vi "TriWave1stEd_YNWang.vi"() -> ()   [LabVIEW 2014]
uses:
  <vilib>/Instr/_visa.llb/VISA Configure Serial Port (Instr).vi
panel:
  in  "Protect scan":bool
  out "Corrent Feedback":dbl
  out "XY Graph":cluster{dbl[], dbl[]}(graph)
  out "Feedback Current":dbl(graph)
  in  "VISA resource name":refnum<visa-resource-name>
  in  "Path":path
  out "Negative Scanning?":bool
  in  "Scan direction":bool
  out "Error":bool
  out "In pause state?":bool
  in  "Pause scan":bool
  in  "Wait before run/s":dbl
  out "Exception Thrown Panel":string
  in  "Emergent STOP":bool
  out "Output V":dbl format="%#_13g"
  in  "End V":dbl format="%#_13g"
  in  "Scan cycle":dbl format="%#_13g"
  out "Volt generator":dbl(graph)
  in  "Step Time/ms":dbl format="%#_13g"
  in  "V per step":dbl format="%#_13g"
  in  "Low V":dbl format="%#_13g"
  in  "High V":dbl format="%#_13g"
  in  "initial V":dbl format="%#_13g"
  # "Pause"
  # "Negative"
  # "Positive"
  # "Continue"
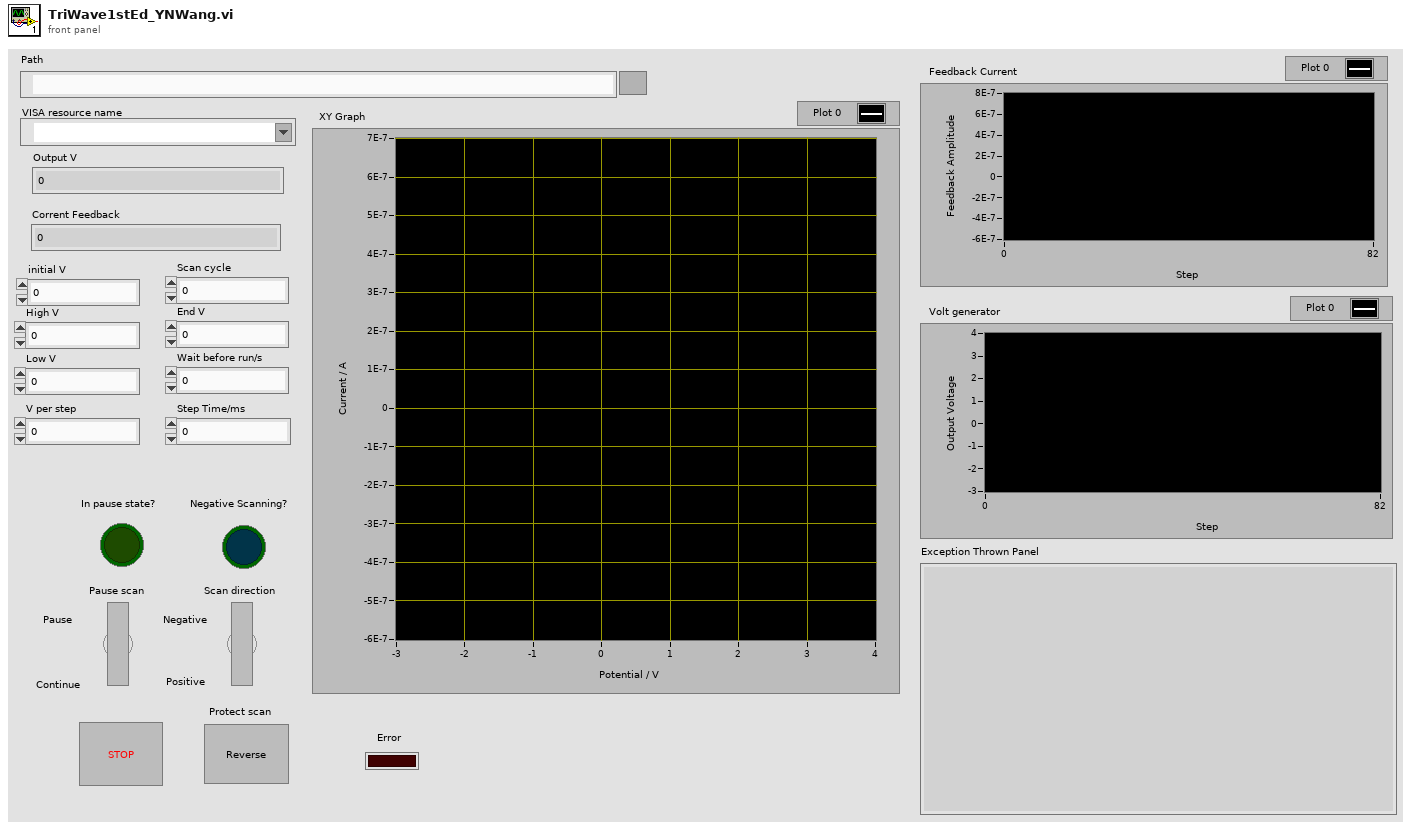
[diagram p1: front panel]
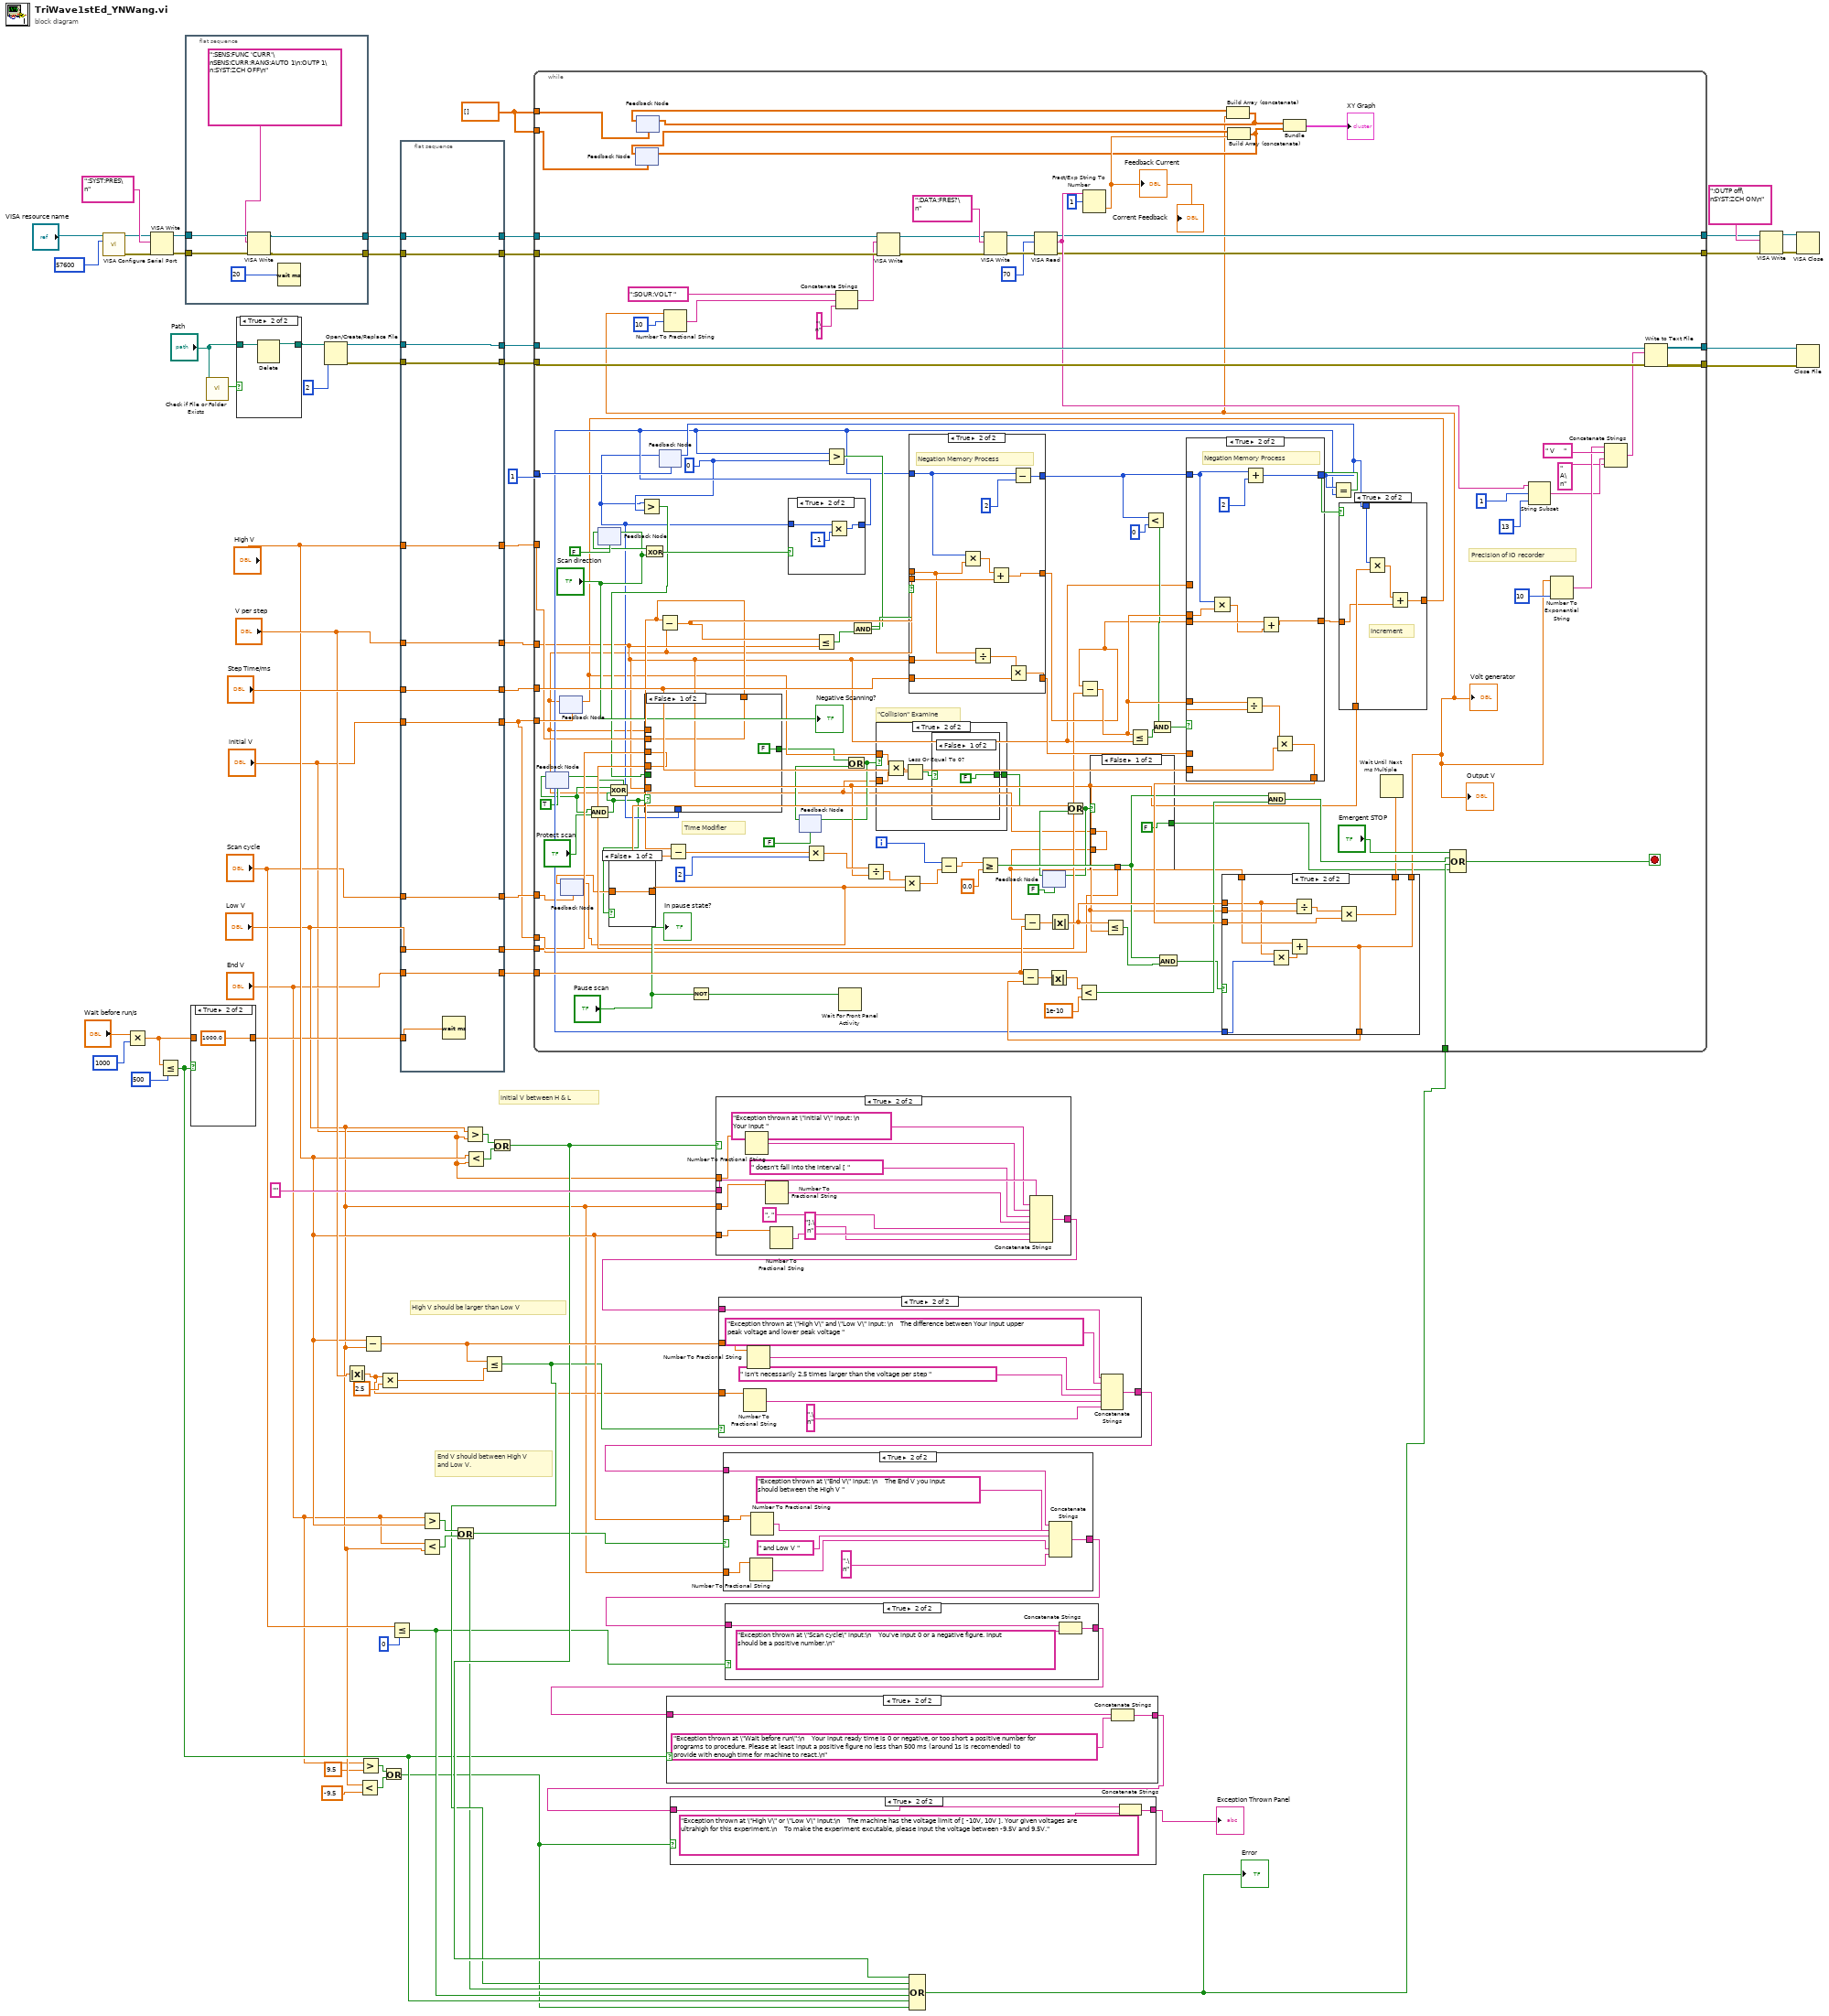
[diagram p0: block diagram]
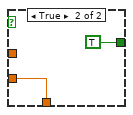
[diagram p10: hidden frame]
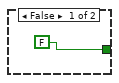
[diagram p11: hidden frame]
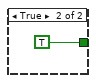
[diagram p12: hidden frame]
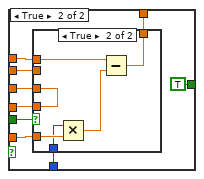
[diagram p13: hidden frame]
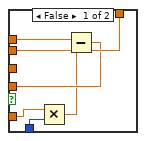
[diagram p14: hidden frame]
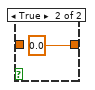
[diagram p15: hidden frame]
diagram:
  w8 = dbl[] []
  # "End V should between High V and Low V."
  # "High V should be larger than Low V"
  # "initial V between H & L"
  n1 = call-poly "VISA Configure Serial Port"("VISA resource name"="VISA resource name", "baud rate (9600)"=57600) -> ("VISA resource name out"=w16:refnum<visa-resource-name>, "error out"=w17:errorcluster)  [unwired: 12 in]
  n2 = Multiply(x="Wait before run/s", y=1000) -> (x*y=w47:dbl)
  n3 = VISA Write(VISA resource name=w16, write buffer=":SYST:PRES\n", error in (no error)=w17) -> (VISA resource name out=w19:refnum<visa-resource-name>, error out=w18:errorcluster)  [unwired: 1 out]
  n4 = Less Or Equal?(x=w47, y=500) -> (x <= y?=w41:bool)
  n5 = flat-sequence {
    tunnel: w19 -> [w80]
    tunnel: w18 -> [w79]
    tunnel: [w77] -> w13
    tunnel: [w76] -> w12
    frame #0 {
      n6 = VISA Write(VISA resource name=w80, write buffer=":SENS:FUNC 'CURR'\nSENS:CURR:RANG:AUTO 1\n:OUTP 1\n:SYST:ZCH OFF\n", error in (no error)=w79) -> (VISA resource name out=w77:refnum<visa-resource-name>, error out=w76:errorcluster)  [unwired: 1 out]
      n7 = Wait (ms)(milliseconds to wait=20) -> ()  [unwired: 1 out]
    }
  }
  n8 = case shown="True" w41 {
    tunnel: [w81 1000.0] -> w48
    tunnel: w47 -> [w81 _]
    frame False {
    }
    frame True {
    }
  }
  n9 = call <vilib>:"Check if File or Folder Exists.vi"("path"="Path") -> ("file or folder exists?"=w30:bool)  [unwired: 8 in, 2 out]
  n10 = case shown="True" w30 {
    tunnel: "Path" -> [w83 w85]
    tunnel: [w83 w84] -> w28
    frame False {
    }
    frame True {
      n11 = Delete(path (use dialog)=w85) -> (deleted path=w84:path)  [unwired: 4 in, 2 out]
    }
  }
  n12 = Open/Create/Replace File(file path (use dialog)=w28, operation (0:open)=2) -> (refnum out=w27:refnum<file>, error out=w25:errorcluster)  [unwired: 4 in, 1 out]
  n13 = Absolute Value(x="V per step") -> (abs(x)=w40:dbl)
  n14 = Less?(x="Low V", y=-9.5) -> (x < y?=w33:bool)
  n15 = Greater?(x="End V", y=9.5) -> (0:w34:bool)
  n16 = Subtract(x="High V", y="Low V") -> (x-y=w61:dbl)
  n17 = Multiply(x=w40, y=2.5) -> (x*y=w60:dbl)
  n18 = Or(x=w34, y=w33) -> (x .or. y?=w32:bool)
  n19 = Less Or Equal?(x="Scan cycle", y=0) -> (x <= y?=w42:bool)
  n20 = flat-sequence {
    tunnel: "High V" -> [w97]
    tunnel: [w97] -> w70
    tunnel: "V per step" -> [w96]
    tunnel: [w96] -> w69
    tunnel: "Step Time/ms" -> [w95]
    tunnel: [w95] -> w67
    tunnel: "initial V" -> [w94]
    tunnel: [w94] -> w1
    tunnel: "Scan cycle" -> [w93]
    tunnel: [w93] -> w66
    tunnel: [w92] -> w65
    tunnel: "Low V" -> [w92]
    tunnel: "End V" -> [w91]
    tunnel: [w91] -> w64
    tunnel: w48 -> [w90]
    tunnel: [w89] -> w26
    tunnel: w27 -> [w89]
    tunnel: [w88] -> w24
    tunnel: w25 -> [w88]
    tunnel: [w87] -> w14
    tunnel: w13 -> [w87]
    tunnel: w12 -> [w86]
    tunnel: [w86] -> w11
    frame #0 {
      n21 = Wait (ms)(milliseconds to wait=w90) -> ()  [unwired: 1 out]
    }
  }
  n22 = Greater?(x="End V", y="High V") -> (0:w56:bool)
  n23 = Less?(x="End V", y="Low V") -> (x < y?=w57:bool)
  n24 = Or(x=w56, y=w57) -> (x .or. y?=w43:bool)
  n25 = Greater?(x="Low V", y="initial V") -> (0:w73:bool)
  n26 = Less?(x="High V", y="initial V") -> (x < y?=w72:bool)
  n27 = Less Or Equal?(x=w61, y=w60) -> (x <= y?=w44:bool)
  n28 = Or(x=w73, y=w72) -> (x .or. y?=w45:bool)
  n29 = case shown="True" w45 {
    tunnel: "" -> [w98 w110]
    tunnel: "initial V" -> [_ w109]
    tunnel: "High V" -> [_ w103]
    tunnel: "Low V" -> [_ w102]
    tunnel: [w98 w99] -> w63
    frame False {
    }
    frame True {
      n30 = Number To Fractional String(number=w109) -> (F-format string=w107:string)  [unwired: 3 in]
      n31 = Number To Fractional String(number=w102) -> (F-format string=w105:string)  [unwired: 3 in]
      n32 = Number To Fractional String(number=w103) -> (F-format string=w101:string)  [unwired: 3 in]
      n33 = Concatenate Strings(w110, "Exception thrown at \"initial V\" input: \n    Your input ", w107, " doesn't fall into the interval [ ", w105, ", ", w101, "].\n") -> (w99:string)
    }
  }
  n34 = case shown="True" w44 {
    tunnel: w63 -> [w111 w119]
    tunnel: w61 -> [_ w118]
    tunnel: w40 -> [_ w115]
    tunnel: [w111 w112] -> w59
    frame False {
    }
    frame True {
      n35 = Number To Fractional String(number=w115) -> (F-format string=w114:string)  [unwired: 3 in]
      n36 = Number To Fractional String(number=w118) -> (F-format string=w117:string)  [unwired: 3 in]
      n37 = Concatenate Strings(w119, "Exception thrown at \"High V\" and \"Low V\" input: \n    The difference between Your input upper peak voltage and lower peak voltage ", w117, " isn't necessarily 2.5 times larger than the voltage per step ", w114, ".\n") -> (w112:string)
    }
  }
  n38 = case shown="True" w43 {
    tunnel: w59 -> [w121 w130]
    tunnel: "High V" -> [_ w128]
    tunnel: "Low V" -> [_ w127]
    tunnel: [w121 w122] -> w54
    frame False {
    }
    frame True {
      n39 = Number To Fractional String(number=w127) -> (F-format string=w124:string)  [unwired: 3 in]
      n40 = Number To Fractional String(number=w128) -> (F-format string=w126:string)  [unwired: 3 in]
      n41 = Concatenate Strings(w130, "Exception thrown at \"End V\" input: \n    The End V you input should between the High V ", w126, " and Low V ", w124, ".\n") -> (w122:string)
    }
  }
  n42 = case shown="True" w42 {
    tunnel: w54 -> [w131 w134]
    tunnel: [w131 w132] -> w46
    frame False {
    }
    frame True {
      n43 = Concatenate Strings(w134, "Exception thrown at \"Scan cycle\" input:\n    You've input 0 or a negative figure. Input should be a positive number.\n") -> (w132:string)
    }
  }
  n44 = case shown="True" w41 {
    tunnel: w46 -> [w135 w138]
    tunnel: [w135 w136] -> w39
    frame False {
    }
    frame True {
      n45 = Concatenate Strings(w138, "Exception thrown at \"Wait before run\":\n    Your input ready time is 0 or negative, or too short a positive number for programs to procedure. Please at least input a positive figure no less than 500 ms (around 1s is recomended) to provide with enough time for machine to react.\n") -> (w136:string)
    }
  }
  n46 = case shown="True" w32 {
    tunnel: w39 -> [w139 w142]
    tunnel: [w139 w140] -> w31
    frame False {
    }
    frame True {
      n47 = Concatenate Strings(w142, "Exception thrown at \"High V\" or \"Low V\" input:\n    The machine has the voltage limit of [ -10V, 10V ]. Your given voltages are ultrahigh for this experiment.\n    To make the experiment excutable, please input the voltage between -9.5V and 9.5V.") -> (w140:string)
    }
  }
  "Exception Thrown Panel" <- w31
  n48 = Compound Arithmetic op=OR(w45, w44, w43, w42, w41, w32) -> (w10:bool)
  "Error" <- w10
  n49 = while {
    tunnel: w1 -> [w255]
    tunnel: 1 -> [w258]
    tunnel: w69 -> [w162]
    tunnel: w70 -> [w173]
    tunnel: w67 -> [w223]
    tunnel: w66 -> [w166]
    tunnel: w64 -> [w222]
    tunnel: w65 -> [w171]
    tunnel: w10 -> [w218]
    tunnel: w26 -> [w211]
    tunnel: w24 -> [w210]
    tunnel: [w209] -> w23
    tunnel: [w208] -> w22
    tunnel: w14 -> [w179]
    tunnel: w11 -> [w178]
    tunnel: w8 -> [w190]
    tunnel: w8 -> [w189]
    tunnel: [w183] -> w4
    tunnel: [w182] -> w3
    tunnel: w1 -> [w146]
    i -> [w244]
    stop <- w221 stop-if-true
    w168 = 0
    # "Precision of IO recorder"
    # "Time Modifier"
    # "\"Collision\" Examine"
    n50 = feedback #1(TRUE) -> (w155:bool)
    n51 = feedback #2(w255) -> (w145:dbl)
    n52 = feedback #3(w166) -> (w165:dbl)
    n53 = And(x=w155, y="Protect scan") -> (x .and. y?=w157:bool)
    n54 = feedback #4(FALSE) -> (w212:bool)
    n55 = feedback-in #4("Scan direction") -> ()
    n56 = Exclusive Or(1:w157, 2:w155) -> (0:w156:bool)
    n57 = feedback-in #1(w156) -> ()
    n58 = case shown="False" w157 {
      tunnel: w165 -> [w296 _]
      tunnel: [w296 0.0] -> w164
      frame False {
      }
      frame True {
      }
    }
    n59 = feedback-in #3(w164) -> ()
    n60 = feedback #5(w189) -> (w187:dbl[])
    n61 = feedback #6(w190) -> (w188:dbl[])
    n62 = Exclusive Or(1:"Scan direction", 2:w212) -> (0:w214:bool)
    n63 = feedback #7(w258) -> (w161:i32)
    n64 = Greater?(x=w161, y=w168) -> (0:w167:bool)
    n65 = case shown="False" w157 {
      tunnel: w173 -> [w274 w282]
      tunnel: [w274 w280] -> w172
      tunnel: w171 -> [w273 w278]
      tunnel: [w273 w279] -> w170
      tunnel: w167 -> [_ w283]
      tunnel: w145 -> [_ w281]
      tunnel: w162 -> [_ w277]
      tunnel: w161 -> [_ w276]
      tunnel: [FALSE TRUE] -> w152
      frame False {
      }
      frame True {
        n66 = case shown="True" w283 {
          tunnel: w282 -> [w289 _]
          tunnel: w281 -> [w285 w291]
          tunnel: [w289 w292] -> w280
          tunnel: [w286 w295] -> w279
          tunnel: w278 -> [_ w295]
          tunnel: w277 -> [w287 w294]
          tunnel: w276 -> [w288 w293]
          frame False {
            n67 = Multiply(x=w287, y=w288) -> (x*y=w284:dbl)
            n68 = Subtract(x=w285, y=w284) -> (x-y=w286:dbl)
          }
          frame True {
            n69 = Multiply(x=w293, y=w294) -> (x*y=w290:dbl)
            n70 = Subtract(x=w291, y=w290) -> (x-y=w292:dbl)
          }
        }
      }
    }
    n71 = Subtract(x=w172, y=w145) -> (x-y=w259:dbl)
    n72 = Subtract(x=w172, y=w170) -> (x-y=w226:dbl)
    n73 = Not(x="Pause scan") -> (.not. x?=w217:bool)
    n74 = case shown="True" w214 {
      tunnel: w161 -> [w298 w301]
      tunnel: [w298 w300] -> w215
      frame False {
      }
      frame True {
        n75 = Multiply(x=w301, y=-1) -> (x*y=w300:i32)
      }
    }
    n76 = feedback #8(FALSE) -> (w153:bool)
    n77 = Multiply(x=w226, y=2) -> (x*y=w225:dbl)
    n78 = Less Or Equal?(x=w259, y=w162) -> (x <= y?=w253:bool)
    n79 = Greater?(x=w215, y=w168) -> (0:w252:bool)
    n80 = Wait For Front Panel Activity(3:w217) -> ()  [unwired: 2 in, 1 out]
    n81 = Or(x=w152, y=w153) -> (x .or. y?=w151:bool)
    n82 = feedback-in #8(w151) -> ()
    n83 = And(x=w252, y=w253) -> (x .and. y?=w254:bool)
    n84 = Divide(x=w225, y=w162) -> (x/y=w245:dbl)
    n85 = Multiply(x=w245, y=w164) -> (x*y=w243:dbl)
    n86 = case shown="True" w254 {
      tunnel: w259 -> [_ w338]
      tunnel: w145 -> [w334 w347]
      tunnel: w223 -> [w336 w346]
      tunnel: w162 -> [_ w345]
      tunnel: [w334 w343] -> w246
      tunnel: [w336 w342] -> w257
      tunnel: w215 -> [w335 w339]
      tunnel: [w335 w337] -> w250
      frame False {
      }
      frame True {
        # "Negation Memory Process"
        n87 = Multiply(x=w339, y=w338) -> (x*y=w340:dbl)
        n88 = Divide(x=w338, y=w345) -> (x/y=w344:dbl)
        n89 = Add(x=w340, y=w347) -> (x+y=w343:dbl)
        n90 = Multiply(x=w344, y=w346) -> (x*y=w342:dbl)
        n91 = Subtract(x=w339, y=2) -> (x-y=w337:i32)
      }
    }
    n92 = Subtract(x=w244, y=w243) -> (x-y=w242:dbl)
    n93 = Greater Or Equal?(x=w242, y=0.0) -> (x >= y?=w231:bool)
    n94 = feedback #9(FALSE) -> (w149:bool)
    n95 = Subtract(x=w246, y=w170) -> (x-y=w256:dbl)
    n96 = Less Or Equal?(x=w256, y=w162) -> (x <= y?=w249:bool)
    n97 = Less?(x=w250, y=0) -> (x < y?=w248:bool)
    n98 = And(x=w248, y=w249) -> (x .and. y?=w247:bool)
    n99 = case shown="True" w247 {
      tunnel: w250 -> [w320 w331]
      tunnel: [w320 w332] -> w227
      tunnel: w256 -> [_ w330]
      tunnel: w246 -> [w319 w324]
      tunnel: [w319 w322] -> w228
      tunnel: w257 -> [w321 w328]
      tunnel: w256 -> [_ w329]
      tunnel: w223 -> [_ w327]
      tunnel: [w321 w325] -> w239
      tunnel: w162 -> [_ _]
      frame False {
      }
      frame True {
        # "Negation Memory Process"
        n100 = Multiply(x=w331, y=w330) -> (x*y=w323:dbl)
        n101 = Divide(x=w329, y=w328) -> (x/y=w326:dbl)
        n102 = Add(x=w331, y=2) -> (x+y=w332:i32)
        n103 = Add(x=w324, y=w323) -> (x+y=w322:dbl)
        n104 = Multiply(x=w326, y=w327) -> (x*y=w325:dbl)
      }
    }
    n105 = feedback-in #7(w227) -> ()
    n106 = Equal?(x=w227, y=w215) -> (x = y?=w229:bool)
    n107 = case shown="True" w229 {
      tunnel: w228 -> [w302 w304]
      tunnel: w227 -> [_ w307]
      tunnel: w162 -> [_ w306]
      tunnel: [w302 w303] -> w154
      frame False {
      }
      frame True {
        # "Increment"
        n108 = Multiply(x=w307, y=w306) -> (x*y=w305:dbl)
        n109 = Add(x=w305, y=w304) -> (x+y=w303:dbl)
      }
    }
    n110 = feedback-in #2(w154) -> ()
    n111 = case shown="True" w151 {
      tunnel: w145 -> [_ w268]
      tunnel: w154 -> [_ w269]
      tunnel: [FALSE w265] -> w148
      frame False {
      }
      frame True {
        n112 = Multiply(x=w269, y=w268) -> (x*y=w267:dbl)
        n113 = Less Or Equal To 0?(x=w267) -> (x <= 0?=w266:bool)
        n114 = case shown="False" w266 {
          tunnel: [FALSE TRUE] -> w265
          frame False {
          }
          frame True {
          }
        }
      }
    }
    n115 = Or(x=w148, y=w149) -> (x .or. y?=w147:bool)
    n116 = feedback-in #9(w147) -> ()
    n117 = case shown="False" w147 {
      tunnel: w146 -> [_ w263]
      tunnel: w145 -> [w261 _]
      tunnel: [w261 w263] -> w144
      tunnel: [FALSE TRUE] -> w143
      frame False {
      }
      frame True {
      }
    }
    n118 = Subtract(x=w144, y=w222) -> (x-y=w240:dbl)
    n119 = Absolute Value(x=w240) -> (abs(x)=w238:dbl)
    n120 = Less Or Equal?(x=w238, y=w162) -> (x <= y?=w232:bool)
    n121 = And(x=w231, y=w232) -> (x .and. y?=w230:bool)
    n122 = case shown="True" w230 {
      tunnel: w144 -> [w308 w314]
      tunnel: w239 -> [w309 w317]
      tunnel: w238 -> [_ w312]
      tunnel: w162 -> [_ w318]
      tunnel: [w309 w315] -> w175
      tunnel: w215 -> [_ w311]
      tunnel: [w308 w310] -> w176
      tunnel: [w308 w310] -> w234
      frame False {
      }
      frame True {
        n123 = Multiply(x=w312, y=w311) -> (x*y=w313:dbl)
        n124 = Add(x=w314, y=w313) -> (x+y=w310:dbl)
        n125 = Divide(x=w312, y=w318) -> (x/y=w316:dbl)
        n126 = Multiply(x=w316, y=w317) -> (x*y=w315:dbl)
      }
    }
    "Volt generator" <- w176
    "Output V" <- w176
    n127 = Number To Fractional String(number=w176, width (-)=10) -> (F-format string=w201:string)  [unwired: 2 in]
    n128 = Concatenate Strings(":SOUR:VOLT ", w201, "\n") -> (w177:string)
    n129 = VISA Write(VISA resource name=w179, write buffer=w177, error in (no error)=w178) -> (VISA resource name out=w181:refnum<visa-resource-name>, error out=w180:errorcluster)  [unwired: 1 out]
    n130 = VISA Write(VISA resource name=w181, write buffer=":DATA:FRES?\n", error in (no error)=w180) -> (VISA resource name out=w197:refnum<visa-resource-name>, error out=w198:errorcluster)  [unwired: 1 out]
    n131 = Subtract(x=w222, y=w234) -> (x-y=w236:dbl)
    n132 = VISA Read(VISA resource name=w197, byte count=u32 70, error in (no error)=w198) -> (VISA resource name out=w183:refnum<visa-resource-name>, read buffer=w195:string, error out=w182:errorcluster)  [unwired: 1 out]
    n133 = Absolute Value(x=w236) -> (abs(x)=w237:dbl)
    n134 = Less?(x=w237, y=1e-10) -> (x < y?=w233:bool)
    n135 = Fract/Exp String To Number(string=w195, offset=1) -> (number=w191:dbl)  [unwired: 2 in, 1 out]
    "Feedback Current" <- w191
    "Corrent Feedback" <- w191
    n136 = Build Array (concatenate)(w188, w176) -> (w185:dbl[])
    n137 = feedback-in #6(w185) -> ()
    n138 = Build Array (concatenate)(w187, w191) -> (w184:dbl[])
    n139 = feedback-in #5(w184) -> ()
    n140 = And(x=w231, y=w233) -> (x .and. y?=w219:bool)
    n141 = Bundle(w185, w184) -> (→"XY Graph":cluster{dbl[], dbl[]})  [unwired: 1 in]
    n142 = Wait Until Next ms Multiple(millisecond multiple=w175) -> ()  [unwired: 1 out]
    n143 = Compound Arithmetic op=OR("Emergent STOP", w219, w218, w143) -> (w221:bool)
    n144 = String Subset(string=w195, offset (0)=1, length (rest)=13 ("length (rest)")) -> (substring=w193:string)
    n145 = Number To Exponential String(number=w176, precision (6)=10) -> (E-format string=w205:string)  [unwired: 2 in]
    n146 = Concatenate Strings(w205, " V     ", w193, " A\n") -> (w206:string)
    n147 = Write to Text File(file (use dialog)=w211, text=w206, error in=w210) -> (refnum out=w209:refnum<file>, error out=w208:errorcluster)  [unwired: 1 in, 1 out]
    "In pause state?" <- "Pause scan"
    "Negative Scanning?" <- "Scan direction"
  }
  n148 = VISA Write(VISA resource name=w4, write buffer=":OUTP off\nSYST:ZCH ON\n", error in (no error)=w3) -> (VISA resource name out=w7:refnum<visa-resource-name>, error out=w6:errorcluster)  [unwired: 1 out]
  n149 = VISA Close(VISA resource name=w7, error in (no error)=w6) -> ()  [unwired: 1 out]
  n150 = Close File(refnum=w23, error in=w22) -> ()  [unwired: 2 out]
